vi "edit io channel.vi"(6 "user event":T2, 8 "error in":errorcluster, 9 "line":T1, 10 "engine configuration in":refnum<class "engine configuration.lvclass">, 11 "Profibus Module configuration in":refnum<class "Profibus Module configuration.lvclass">) -> (0 "error out":errorcluster, 2 "engine configuration out":refnum<class "engine configuration.lvclass">, 3 "Profibus Module configuration out":refnum<class "Profibus Module configuration.lvclass">)   [LabVIEW 2013, in "Profibus Module editor node.lvclass"]
uses:
  Profibus Module editor node.lvclass
  <vilib>/NI/Configuration Framework/Node/UserEventRef.ctl
  <vilib>/NI/Configuration Framework/Controls/EventCluster.ctl
  <vilib>/NI/Module Execution Interface/Engine Configuration/engine configuration.lvclass
  configuration/Profibus Module configuration.lvclass
  table line.ctl
  channel/Profibus channel.lvclass
  <vilib>/NI/Configuration Framework/serializable configuration/NISE_CEF_serializable configuration.lvclass/NISE_CEF_serializable configuration.ctl
  <vilib>/NI/Tag Bus/tag/tag descriptor.lvclass/tag descriptor.ctl
  <vilib>/Utility/LVClass/Get LV Class Name.vi
  <vilib>/NI/Configuration Framework/error generator/NISE_error generator.vi
  <vilib>/NI/Configuration Framework/NISE_CEF_TreeControl.lvlib
  <vilib>/NI/Tag Bus/tag/tag descriptor.lvclass
  <vilib>/NI/Configuration Framework/serializable configuration/NISE_CEF_serializable configuration.lvclass
  <vilib>/NI/Configuration Framework/Node/NISE_CEF_Node.lvclass
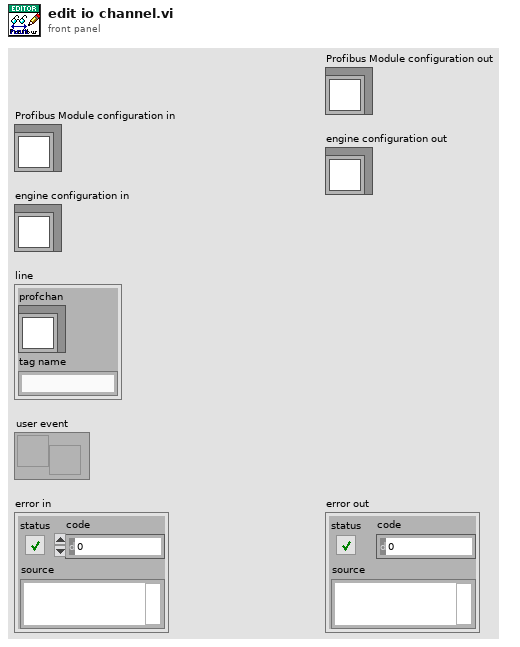
[diagram p1: front panel]
types:
  T1 = typedef "Profibus Module editor node.lvclass/table line.ctl" = cluster{"profchan":refnum<class "Profibus channel.lvclass">, "tag name":string}
  T2 = typedef "NISE_CEF_Node.lvclass/UserEventRef.ctl" = refnum<user-event>
  T3 = typedef "NISE_CEF_TreeControl.lvlib/EventCluster.ctl" = cluster{"command":string, "data":string}
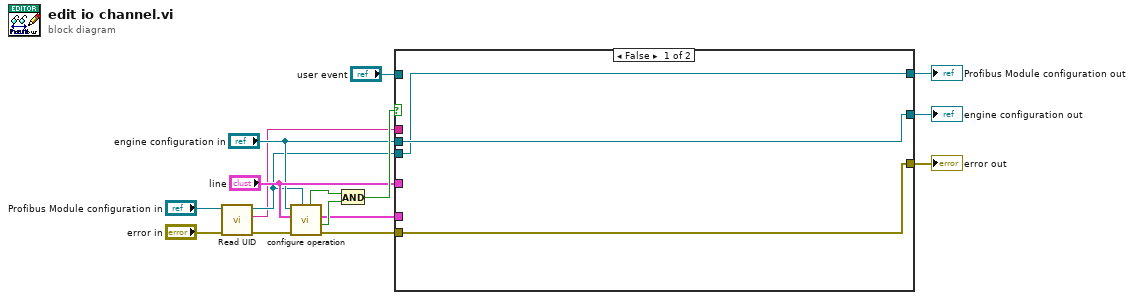
[diagram p0: block diagram]
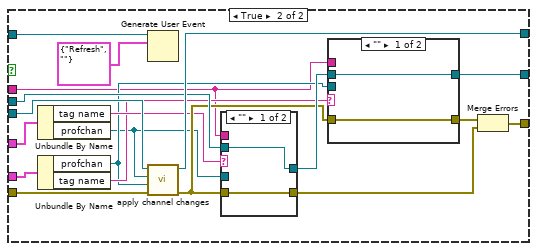
[diagram p2: hidden frame]
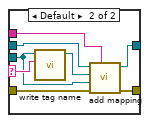
[diagram p3: hidden frame]
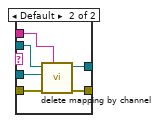
[diagram p4: hidden frame]
diagram:
  n1 = call <vilib>:"Read UID.vi"("error in"="error in", "configuration in"="Profibus Module configuration in") -> ("error out"=w4:errorcluster, "instance id"=w1:string, "configuration out"=w2:refnum<class "Profibus Module configuration.lvclass">)  [unwired: 7 in]
  n2 = call "configure operation.vi"("owner ID"=w2, "error in"=w4, "line item in"="line", "engine configuration in"="engine configuration in") -> ("error out"=w8:errorcluster, "success"=w12:bool, "line item out"=w9:T1, "changed"=w11:bool)  [unwired: 4 in]
  n3 = And(x=w11, y=w12) -> (x .and. y?=w13:bool)
  n4 = case shown="False" w13 {
    tunnel: [w18 w28] -> w6
    tunnel: [w19 w26] -> w15
    tunnel: "engine configuration in" -> [w19 w27]
    tunnel: w8 -> [w18 w36]
    tunnel: w9 -> [_ w33]
    tunnel: "line" -> [_ w37]
    tunnel: w2 -> [w17 w38]
    tunnel: [w17 w32] -> w14
    tunnel: w1 -> [_ w20]
    tunnel: "user event" -> [_ w34]
    frame False {
    }
    frame True {
      n5 = Unbundle By Name(w37) -> ("tag name"=w24:string, "profchan"=w21:refnum<class "Profibus channel.lvclass">)
      n6 = Unbundle By Name(w33) -> ("profchan"=w22:refnum<class "Profibus channel.lvclass">, "tag name"=w23:string)
      n7 = Generate User Event(user event=w34, event data cluster=T3 {"command"="Refresh", "data"=""} ("event data")) -> ()  [unwired: 2 in, 2 out]
      n8 = call "apply channel changes.vi"("error in"=w36, "new"=w22, "old"=w21, "Profibus Module configuration in"=w38) -> ("error out"=w25:errorcluster, "Profibus Module configuration out"=w32:refnum<class "Profibus Module configuration.lvclass">)  [unwired: 6 in]
      n9 = case shown="\"\"" w24 {
        tunnel: w20 -> [_ w56]
        tunnel: w27 -> [w50 w55]
        tunnel: [w50 w54] -> w29
        tunnel: [w49 w53] -> w30
        tunnel: w25 -> [w49 w52]
        tunnel: w21 -> [_ w51]
        frame "" {
        }
        frame Default {
          n10 = call <vilib>:"delete mapping by channel.vi"("owner ID"=w56, "error in"=w52, "channel"=w51, "engine configuration in"=w55) -> ("error out"=w53:errorcluster, "engine configuration out"=w54:refnum<class "engine configuration.lvclass">)  [unwired: 6 in]
        }
      }
      n11 = case shown="\"\"" w23 {
        selector: w23 -> [_ w42]
        tunnel: w29 -> [w40 w48]
        tunnel: [w40 w47] -> w26
        tunnel: [w39 w46] -> w31
        tunnel: w25 -> [w39 w45]
        tunnel: w20 -> [_ w44]
        tunnel: w22 -> [_ w41]
        frame "" {
        }
        frame Default {
          n12 = call <vilib>:"write tag name.vi"("name"=w42, "system tag in"=w41) -> ("system tag out"=w43:refnum<class "Profibus channel.lvclass">)  [unwired: 8 in, 1 out]
          n13 = call <vilib>:"add mapping.vi"("owner ID"=w44, "error in"=w45, "channel"=w41, "tag descriptor"=w43, "engine configuration"=w48) -> ("error out"=w46:errorcluster, "engine configuration out"=w47:refnum<class "engine configuration.lvclass">)  [unwired: 5 in]
        }
      }
      n14 = Merge Errors(w31, w30) -> (w28:errorcluster)
    }
  }
  "engine configuration out" <- w15
  "Profibus Module configuration out" <- w14
  "error out" <- w6
